vi "varXNode_Mutate_1_0_0_4.vi"(8 "error in (no error)":errorcluster, 9 "Replies in":string[](array[string]), 10 "Version":T1, 11 "Old State":variant) -> (0 "error out":errorcluster, 1 "Replies out":string[](array[string]), 2 "Version Out":T1, 3 "New State":variant)   [LabVIEW 2020, in "varXNode.xnode"]
uses:
  <vilib>/variable/varXNode.llb/varXNode.xnode
  <vilib>/XNodeSupport/XNodeVersion.ctl
  <vilib>/XNodeSupport/XNodeUShort.ctl
  <vilib>/variable/varXNode.llb/varXNode_old_1_0_0_3.ctl
  <vilib>/variable/varXNode.llb/varXNode_old_1_0_0_4.ctl
  <vilib>/XNodeSupport/NI_XNodeSupport.lvlib
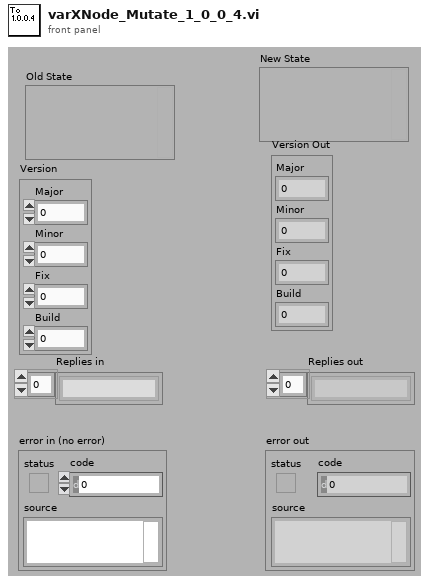
[diagram p1: front panel]
types:
  T1 = typedef "NI_XNodeSupport.lvlib/XNodeVersion.ctl" = cluster{"Major":T2, "Minor":T2, "Fix":T2, "Build":T2}
  T2 = typedef "NI_XNodeSupport.lvlib/XNodeUShort.ctl" = u16
  T3 = typedef "varXNode.xnode/varXNode_old_1_0_0_4.ctl" = cluster{"Write":bool, "ShowTimestamp":bool, "CachedName":string, "CachedTypeDesc":i16[], "CachedFeaturePacks":string[], "Custom Rule":string, "ProjectPath":string, "Bad Code":bool, "ContextName":string}
  T4 = typedef "varXNode.xnode/varXNode_old_1_0_0_3.ctl" = cluster{"Write":bool, "ShowTimestamp":bool, "CachedName":string, "CachedTypeDesc":i16[], "CachedFeaturePacks":string[], "Custom Rule":string, "ProjectPath":string, "Bad Code":bool}
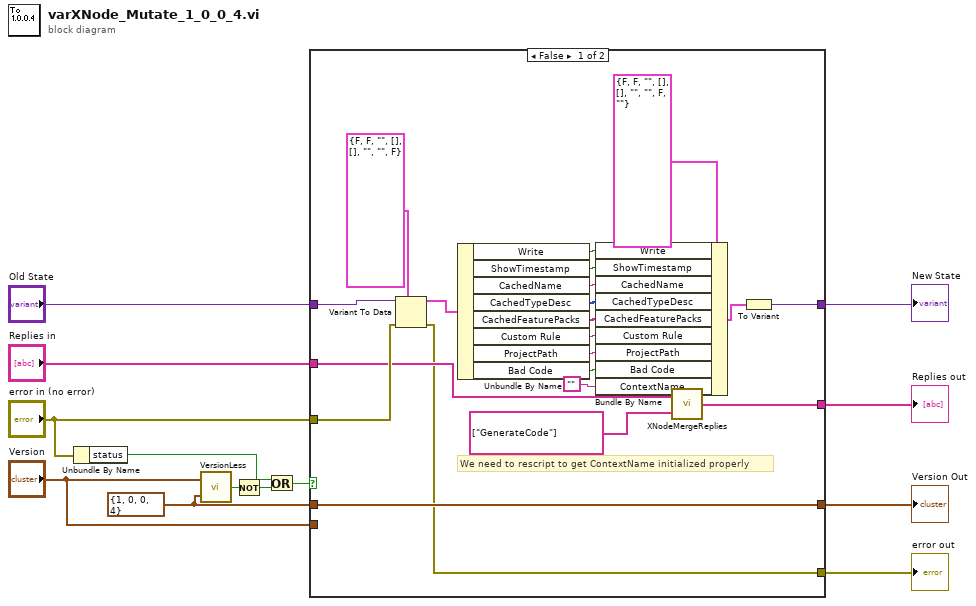
[diagram p0: block diagram]
diagram:
  w12 = T1 {"Major"=1, "Minor"=0, "Fix"=0, "Build"=4} ("y")
  n1 = Unbundle By Name("error in (no error)") -> ("status"=w4:bool)
  n2 = call <vilib>:"VersionLess.vi"("y"=w12, "x"="Version") -> ("x < y?"=w13:bool)
  n3 = Not(x=w13) -> (.not. x?=w3:bool)
  n4 = Or(x=w4, y=w3) -> (x .or. y?=w6:bool)
  n5 = case shown="False" w6 {
    tunnel: w12 -> [w34 _]
    tunnel: [w22 w38] -> w11
    tunnel: "Old State" -> [w33 w38]
    tunnel: [w34 w37] -> w9
    tunnel: "Version" -> [_ w37]
    tunnel: [w18 w36] -> w7
    tunnel: "error in (no error)" -> [w32 w36]
    tunnel: [w19 w35] -> w2
    tunnel: "Replies in" -> [w21 w35]
    frame False {
      # "We need to rescript to get ContextName initialized properly"
      n6 = Variant To Data(error in=w32, type=T4 {"Write"=FALSE, "ShowTimestamp"=FALSE, "CachedName"="", "CachedTypeDesc"=[], "CachedFeaturePacks"=[], "Custom Rule"="", "ProjectPath"="", "Bad Code"=FALSE} ("State"), Variant=w33) -> (data=w31:T4, error out=w18:errorcluster)
      n7 = Unbundle By Name(w31) -> ("Write"=w30:bool, "ShowTimestamp"=w29:bool, "CachedName"=w28:string, "CachedTypeDesc"=w27:i16[], "CachedFeaturePacks"=w26:string[], "Custom Rule"=w25:string, "ProjectPath"=w24:string, "Bad Code"=w16:bool)
      n8 = Bundle By Name(cluster=T3 {"Write"=FALSE, "ShowTimestamp"=FALSE, "CachedName"="", "CachedTypeDesc"=[], "CachedFeaturePacks"=[], "Custom Rule"="", "ProjectPath"="", "Bad Code"=FALSE, "ContextName"=""} ("State"), "Write"=w30, "ShowTimestamp"=w29, "CachedName"=w28, "CachedTypeDesc"=w27, "CachedFeaturePacks"=w26, "Custom Rule"=w25, "ProjectPath"=w24, "Bad Code"=w16, "ContextName"="") -> (w23:T3)
      n9 = call <vilib>:"XNodeMergeReplies.vi"("New Replies"=string[] ["GenerateCode"] ("Replies out"), "Old Replies"=w21) -> ("Merged Replies"=w19:string[])
      n10 = To Variant(anything=w23) -> (Variant=w22:variant)
    }
    frame True {
      # "Either there was an error in,\nor the version is not less than 1.0.0.2.\nPass input values out."
    }
  }
  "New State" <- w11
  "Version Out" <- w9
  "error out" <- w7
  "Replies out" <- w2
